vi "Send Sample Command.vi"(8 "error in (no error)":errorcluster, 11 "Serial Device":refnum<class "Serial Device.lvclass">) -> (0 "error out":errorcluster, 2 "Response to Sample Command":string, 3 "Serial Device Out":refnum<class "Serial Device.lvclass">)   [LabVIEW 2017, in "Serial Device.lvclass"]
uses:
  Serial Device.lvclass
  Get Serial Port.vi
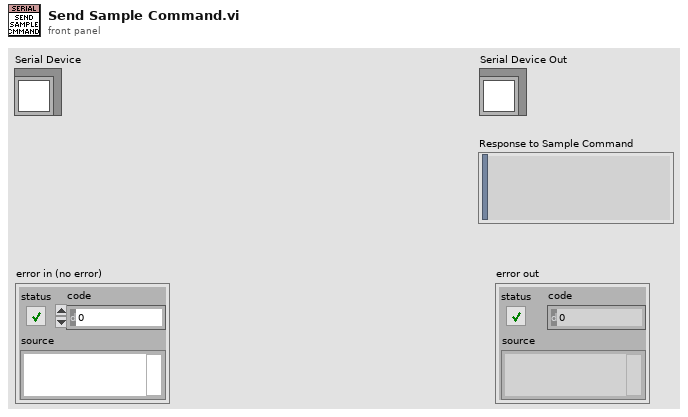
[diagram p1: front panel]
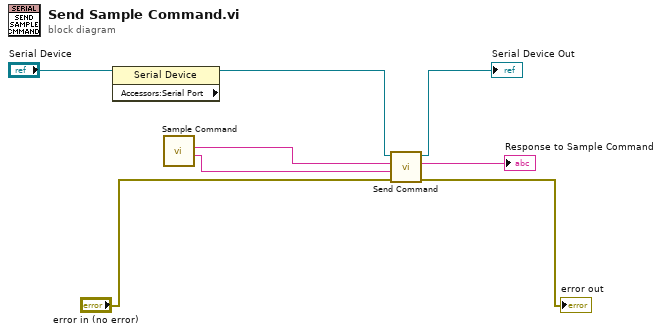
[diagram p0: block diagram]
diagram:
  n1 = property class="Serial Device" props=["Accessors:Serial Port"](reference="Serial Device") -> (reference out=w2:refnum<class "Serial Device.lvclass">)  [unwired: 1 in, 2 out]
  n2 = call "Sample Command.vi"() -> ("Expected Response"=w5:string, "Sample Command"=w7:string)  [unwired: 10 in]
  n3 = call-dynamic "Send Command.vi"("error in (no error)"="error in (no error)", "Expected Response"=w5, "Command"=w7, "Serial Device"=w2) -> ("error out"=→"error out":errorcluster, "read buffer"=→"Response to Sample Command":string, "Serial Device Out"=→"Serial Device Out":refnum<class "Serial Device.lvclass">)  [unwired: 5 in]
